vi "GetWaitValues.vi"(8 "error in (no error)":errorcluster caption="entrée d'erreur (pas d'erreur)", 11 "BaseDevice en entrée":refnum<class "BaseDevice.lvclass"> caption="DNL_LabVIEW Object in") -> (0 "error out":errorcluster caption="sortie d'erreur", 1 "Afterwait(ms)":u32, 2 "Beforewait(ms)":u32, 3 "BaseDevice en sortie":refnum<class "BaseDevice.lvclass"> caption="DNL_LabVIEW Object out", 4 "SynchToClk(ms)":i32)   [LabVIEW 2019, in "BaseDevice.lvclass"]
uses:
  BaseDevice.lvclass
  BaseDevice.lvclass/BaseDevice.ctl
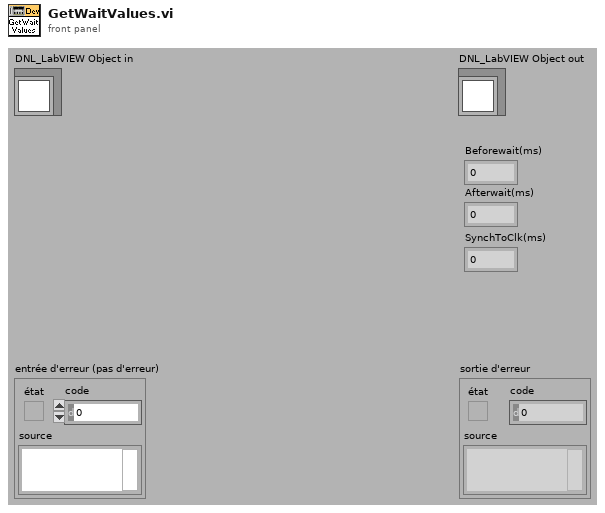
[diagram p1: front panel]
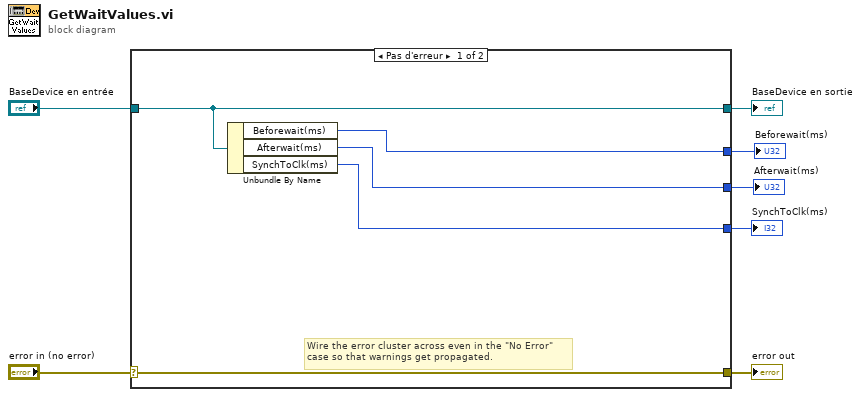
[diagram p0: block diagram]
diagram:
  n1 = case shown="Pas d'erreur" "error in (no error)" {
    selector: "error in (no error)" -> [w12 w14]
    tunnel: [w12 w14] -> w6
    tunnel: [w11 w13] -> w4
    tunnel: "BaseDevice en entrée" -> [w11 w13]
    tunnel: [w10 _] -> w3
    tunnel: [w9 _] -> w2
    tunnel: [w8 _] -> w1
    frame No Error {
      # "Wire the error cluster across even in the \"No Error\"\ncase so that warnings get propagated."
      n2 = Unbundle By Name(w11) -> ("Beforewait(ms)"=w10:u32, "Afterwait(ms)"=w9:u32, "SynchToClk(ms)"=w8:i32)
    }
    frame Error {
    }
  }
  "error out" <- w6
  "BaseDevice en sortie" <- w4
  "Beforewait(ms)" <- w3
  "Afterwait(ms)" <- w2
  "SynchToClk(ms)" <- w1
